vi "Sensor Data (Scope).vi"(8 "error in (no error)":errorcluster, 9 "Temp. Unit(0:K,1:C)":i32, 11 "VISA resource name":refnum<visa-resource-name>) -> (0 "error out":errorcluster, 1 "Data B":dbl, 2 "Data A":dbl, 3 "VISA resource name out":refnum<visa-resource-name>)   [LabVIEW 2015]
doc: "Reads and returns multiple sensor readings from the instrument. Control over interval between readings is also provided."
uses:
  Lake Shore 335.lvlib
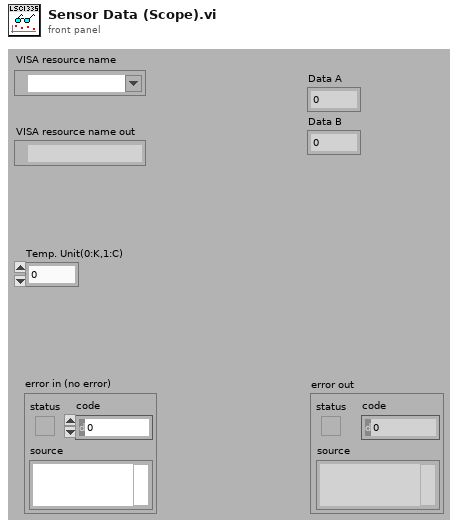
[diagram p1: front panel]
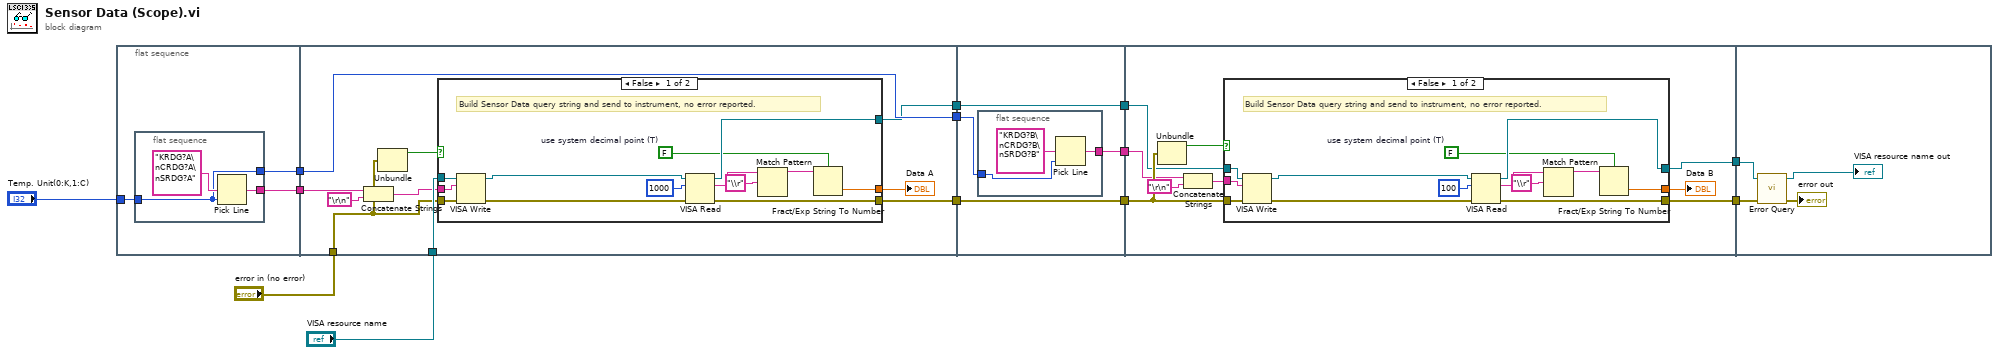
[diagram p0: block diagram]
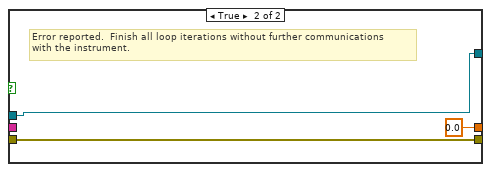
[diagram p2: hidden frame]
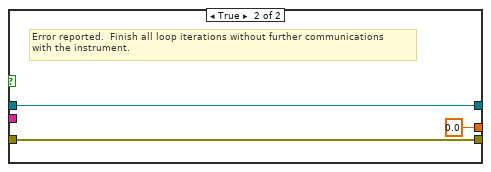
[diagram p3: hidden frame]
diagram:
  n1 = flat-sequence {
    tunnel: "Temp. Unit(0:K,1:C)" -> [w16]
    tunnel: [w15] -> w13
    tunnel: [w14] -> w4
    tunnel: w13 -> [w29]
    tunnel: "VISA resource name" -> [w25]
    tunnel: [w23] -> w10
    tunnel: [w24] -> w9
    tunnel: "error in (no error)" -> [w21]
    tunnel: [w27] -> w5
    tunnel: w4 -> [w27]
    tunnel: [w49] -> w11
    tunnel: w10 -> [w49]
    tunnel: w9 -> [w48]
    tunnel: [w48] -> w8
    tunnel: w5 -> [w47]
    tunnel: [w46] -> w2
    tunnel: w11 -> [w59]
    tunnel: w8 -> [w61]
    tunnel: [w58] -> w3
    tunnel: w2 -> [w54]
    tunnel: [w57] -> w1
    tunnel: w3 -> [w78]
    tunnel: w1 -> [w79]
    frame #0 {
      n2 = flat-sequence {
        tunnel: [w18] -> w15
        tunnel: w16 -> [w17]
        tunnel: [w17] -> w14
        frame #0 {
          n3 = Pick Line(multi-line string="KRDG?A\nCRDG?A\nSRDG?A", line index=w17) -> (output string=w18:string)  [unwired: 1 in]
        }
      }
    }
    frame #1 {
      n4 = Concatenate Strings(w29, "\r\n") -> (w20:string)
      n5 = Unbundle(w21) -> ("status"=w26:bool)  [unwired: 2 out]
      n6 = case shown="False" w26 {
        tunnel: w25 -> [w42 w45]
        tunnel: [w41 w45] -> w23
        tunnel: [w33 0.0] -> w22
        tunnel: w21 -> [w32 w44]
        tunnel: [w31 w44] -> w24
        tunnel: w20 -> [w30 _]
        frame False {
          w35 = FALSE  # use system decimal point (T)
          # "Build Sensor Data query string and send to instrument, no error reported."
          n7 = VISA Write(VISA resource name=w42, write buffer=w30, error in (no error)=w32) -> (VISA resource name out=w37:refnum<visa-resource-name>, error out=w36:errorcluster)  [unwired: 1 out]
          n8 = VISA Read(VISA resource name=w37, byte count=1000, error in (no error)=w36) -> (VISA resource name out=w41:refnum<visa-resource-name>, read buffer=w39:string, error out=w31:errorcluster)  [unwired: 1 out]
          n9 = Match Pattern(string=w39, regular expression="\\r") -> (before substring=w34:string)  [unwired: 1 in, 3 out]
          n10 = Fract/Exp String To Number(use system decimal point (T)=w35, string=w34) -> (number=w33:dbl)  [unwired: 2 in, 1 out]
        }
        frame True {
          # "Error reported.  Finish all loop iterations without further communications\nwith the instrument."
        }
      }
      "Data A" <- w22
    }
    frame #2 {
      n11 = flat-sequence {
        tunnel: [w51] -> w46
        tunnel: w47 -> [w50]
        frame #0 {
          n12 = Pick Line(multi-line string="KRDG?B\nCRDG?B\nSRDG?B", line index=w50) -> (output string=w51:string)  [unwired: 1 in]
        }
      }
    }
    frame #3 {
      n13 = Unbundle(w61) -> ("status"=w60:bool)  [unwired: 2 out]
      n14 = Concatenate Strings(w54, "\r\n") -> (w53:string)
      n15 = case shown="False" w60 {
        tunnel: w59 -> [w74 w77]
        tunnel: [w73 w77] -> w57
        tunnel: [w65 0.0] -> w56
        tunnel: w61 -> [w64 w76]
        tunnel: [w63 w76] -> w58
        tunnel: w53 -> [w62 _]
        frame False {
          w67 = FALSE  # use system decimal point (T)
          # "Build Sensor Data query string and send to instrument, no error reported."
          n16 = VISA Write(VISA resource name=w74, write buffer=w62, error in (no error)=w64) -> (VISA resource name out=w69:refnum<visa-resource-name>, error out=w68:errorcluster)  [unwired: 1 out]
          n17 = VISA Read(VISA resource name=w69, byte count=100, error in (no error)=w68) -> (VISA resource name out=w73:refnum<visa-resource-name>, read buffer=w71:string, error out=w63:errorcluster)  [unwired: 1 out]
          n18 = Match Pattern(string=w71, regular expression="\\r") -> (before substring=w66:string)  [unwired: 1 in, 3 out]
          n19 = Fract/Exp String To Number(use system decimal point (T)=w67, string=w66) -> (number=w65:dbl)  [unwired: 2 in, 1 out]
        }
        frame True {
          # "Error reported.  Finish all loop iterations without further communications\nwith the instrument."
        }
      }
      "Data B" <- w56
    }
    frame #4 {
      n20 = call "Error Query.vi"("error in (no error)"=w78, "VISA resource name"=w79) -> ("error out"=→"error out":errorcluster, "VISA resource name out"=→"VISA resource name out":refnum<visa-resource-name>)  [unwired: 7 in, 1 out]
    }
  }
